vi "GetLSEEstimate.vi"(8 "error in":errorcluster, 9 "NetworkData":T1, 10 "lsecon":T2={"NoiseVariance"=0.001, "IEEESystem"=5, "PMULocations"=[1], "Vindex"=0, "Iindex"=3, "DynamicRef"=""}, 11 "measure_input":cdb[][](array[numeric])) -> (0 "error out":errorcluster, 2 "test_array":dbl[](array[numeric]), 3 "Vestimate":cdb[](array[numeric]))   [LabVIEW 2017, in "AppPlugins.lvlib" / "LSEPlugin.lvclass"]
uses:
  LSEPlugin.lvclass
  Typedefs/LSEConfig.ctl
  Typedefs/Network.ctl
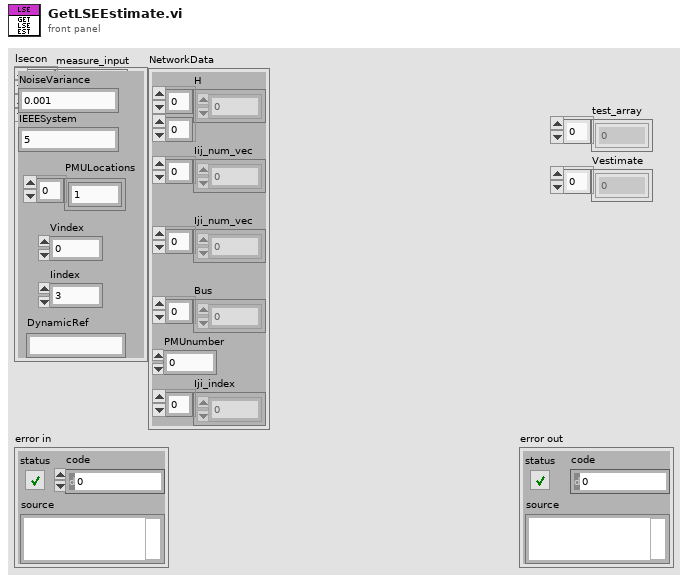
[diagram p1: front panel]
types:
  T1 = typedef "AppPlugins.lvlib/LSEPlugin.lvclass/Network.ctl" = cluster{"H":dbl[][], "Iij_num_vec":dbl[], "Iji_num_vec":dbl[], "Bus":dbl[], "PMUnumber":i32, "Iji_index":i32[]}
  T2 = typedef "AppPlugins.lvlib/LSEPlugin.lvclass/LSEConfig.ctl" = cluster{"NoiseVariance":dbl, "IEEESystem":u32, "PMULocations":u32[], "Vindex":i32, "Iindex":i32, "DynamicRef":string}
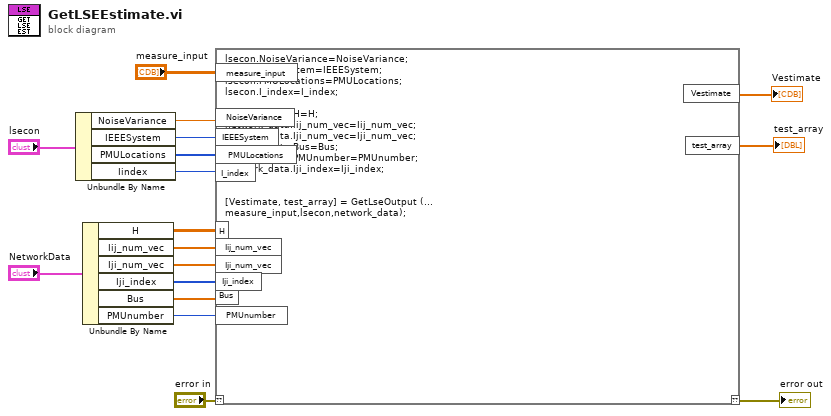
[diagram p0: block diagram]
diagram:
  n1 = Unbundle By Name("lsecon") -> ("NoiseVariance"=w12:dbl, "IEEESystem"=w11:u32, "PMULocations"=w10:u32[], "Iindex"=w1:i32)
  n2 = Unbundle By Name("NetworkData") -> ("H"=w9:dbl[][], "Iij_num_vec"=w8:dbl[], "Iji_num_vec"=w7:dbl[], "Iji_index"=w4:i32[], "Bus"=w3:dbl[], "PMUnumber"=w2:i32)
  n3 = script code="lsecon.NoiseVariance=NoiseVariance; \nlsecon.IEEESystem=IEEESystem;\nlsecon.PMULocations=PMULocations;\nlsecon.I_index=I_index;\n\nnetwork_data.H=H;\nnetwork_data.Iij_num_vec=Iij_num_vec;\nnetwork_data.Iji_num_vec=Iji_num_vec;\nnetwork_data.Bus=Bus;\nnetwork_data.PMUnumber=PMUnumber;\nnetwork_data.Iji_index=Iji_index;\n\n\n[Vestimate, test_array] = GetLseOutput (...\nmeasure_input,lsecon,network_data);"("??"="error in", "measure_input"="measure_input", "NoiseVariance"=w12, "IEEESystem"=w11, "PMULocations"=w10, "H"=w9, "Iij_num_vec"=w8, "Iji_num_vec"=w7, "Bus"=w3, "PMUnumber"=w2, "Iji_index"=w4, "I_index"=w1) -> ("??"=→"error out":errorcluster, "test_array"=→"test_array":dbl[], "Vestimate"=→"Vestimate":cdb[])
